vi "TL_stop_scan.vi"(5 "queue DAQ":refnum<queue>, 7 "queue sCMOS":refnum<queue>, 8 "error in":errorcluster, 9 "BF?":bool, 10 "queue piezo":refnum<queue>, 11 "queue ASI stage":refnum<queue>) -> (0 "error out":errorcluster)   [LabVIEW 2015]
uses:
  CONTROLS/Q_ASI_stage_element.ctl
  CONTROLS/Q_DAQ_element.ctl
  CONTROLS/Q_MCL_piezo_element.ctl
  CONTROLS/Q_camera_element.ctl
  GLOBAL/Global_DAQ.vi
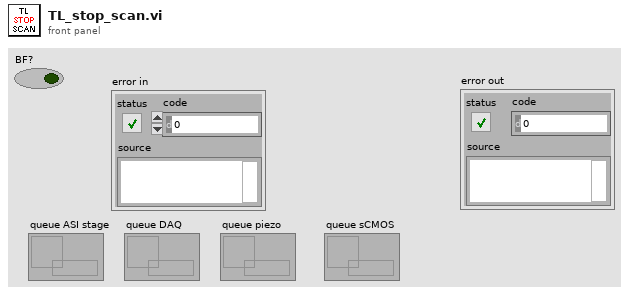
[diagram p1: front panel]
types:
  T1 = typedef "Q_camera_element.ctl" = cluster{"variant":variant, "Instruction":enum16{"CAMERA_idle", "CAMERA_initialize", "CAMERA_error", "CAMERA_security_stop", "CAMERA_not_acquiring", "CAMERA_acquiring", "CAMERA_start_acquiring", "CAMERA_stop_acquiring", "CAMERA_change_exposure", "CAMERA_define_ROI", "CAMERA_cooler", "CAMERA_acquire_movie", "CAMERA_init_scan", "CAMERA_check_new_scan_image", "CAMERA_close_scan", "CAMERA_init_merFISH", "CAMERA_start_acquiring_merFISH", "CAMERA_close_scan_merFISH", "CAMERA_close_merFISH", "CAMERA_init_TL", "CAMERA_start_acquiring_TL", "CAMERA_stop_acquiring_TL", "CAMERA_close_TL", "CAMERA_STOP"}}
  T2 = typedef "Q_MCL_piezo_element.ctl" = cluster{"variant":variant, "Instruction":enum16{"Piezo_idle", "Piezo_initialize", "Piezo_error", "Piezo_security_stop", "Piezo_read_z", "Piezo_move_z", "Piezo_keyboard_move", "Piezo_close_autofocus_calibration_ramp", "Piezo_change_init_state", "Piezo_init_autofocus", "Piezo_init_autofocus_merFISH_TL", "Piezo_autofocus", "Piezo_autofocus_merFISH_TL", "Piezo_stop_autofocus", "Piezo_stop_autofocus_merFISH_TL", "Piezo_autofocus_lost", "Piezo_resume_autofocus_merFISH_TL", "Piezo_check_z_position_merFISH_TL", "Piezo_init_ramp", "Piezo_move_z_ramp", "Piezo_close_ramp", "Piezo_close_merFISH", "Piezo_init_TL", "Piezo_close_ramp_TL", "Piezo_close_TL", "Piezo_stop"}}
  T3 = typedef "Q_ASI_stage_element.ctl" = cluster{"variant":variant, "Instruction":enum16{"ASI_idle", "ASI_initialize", "ASI_error", "ASI_security_stop", "ASI_read_XYZ", "ASI_up", "ASI_down", "ASI_left", "ASI_right", "ASI_save_XY", "ASI_move_to_XY", "ASI_brightfield", "ASI_init_scan", "ASI_init_merFISH", "ASI_move_to_XY_merFISH", "ASI_move_to_Z_merFISH", "ASI_init_autofocus_search_merFISH", "ASI_close_autofocus_search_merFISH", "ASI_adjust_piezo_autofocus_merFISH", "ASI_set_piezo_autofocus_to_reference_position_merFISH_TL", "ASI_close_merFISH", "ASI_init_TL", "ASI_move_mosaic_TL", "ASI_brightfield_TL", "ASI_close_TL", "ASI_stop"}}
  T4 = typedef "Q_DAQ_element.ctl" = cluster{"variant":variant, "Instruction":enum16{"DAQ_idle", "DAQ_initialize", "DAQ_error", "DAQ_security_stop", "DAQ_start_QPD", "DAQ_change_QPD_display", "DAQ_read_display_QPD_signal", "DAQ_QPD_init_autofocus", "DAQ_read_display_send_QPD_signal", "DAQ_close_autofocus_calibration_ramp", "DAQ_close_autofocus", "DAQ_405", "DAQ_488", "DAQ_561", "DAQ_641", "DAQ_zero_all", "DAQ_init_single_scan", "DAQ_single_scan", "DAQ_two_way_valve", "DAQ_init_merFISH", "DAQ_scan_merFISH", "DAQ_photobleaching_merFISH", "DAQ_close_merFISH", "DAQ_init_TL", "DAQ_synchro_TL", "DAQ_close_task_TL", "DAQ_close_TL", "DAQ_stop"}}
  T5 = enum16{"DAQ_idle", "DAQ_initialize", "DAQ_error", "DAQ_security_stop", "DAQ_start_QPD", "DAQ_change_QPD_display", "DAQ_read_display_QPD_signal", "DAQ_QPD_init_autofocus", "DAQ_read_display_send_QPD_signal", "DAQ_close_autofocus_calibration_ramp", "DAQ_close_autofocus", "DAQ_405", "DAQ_488", "DAQ_561", "DAQ_641", "DAQ_zero_all", "DAQ_init_single_scan", "DAQ_single_scan", "DAQ_two_way_valve", "DAQ_init_merFISH", "DAQ_scan_merFISH", "DAQ_photobleaching_merFISH", "DAQ_close_merFISH", "DAQ_init_TL", "DAQ_synchro_TL", "DAQ_close_task_TL", "DAQ_close_TL", "DAQ_stop"}
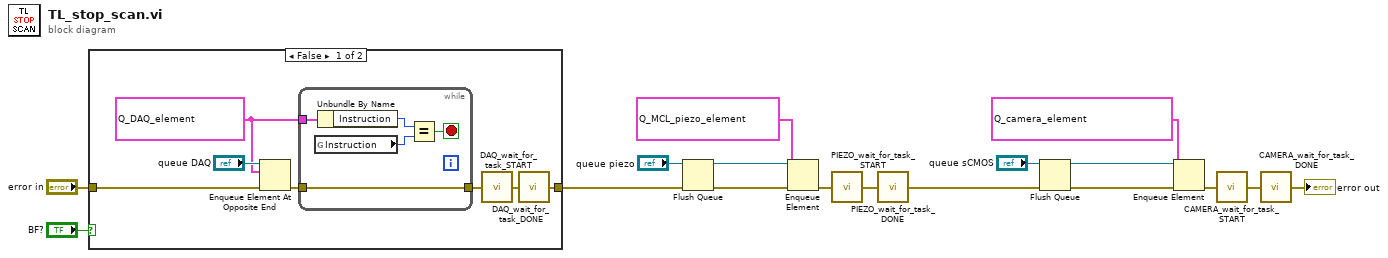
[diagram p0: block diagram]
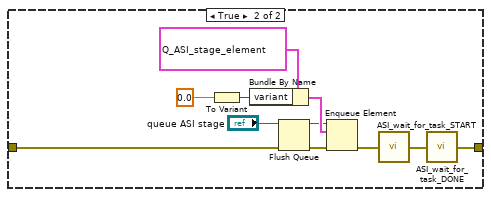
[diagram p2: hidden frame]
diagram:
  n1 = case shown="False" "BF?" {
    tunnel: "error in" -> [w24 w33]
    tunnel: [w22 w37] -> w14
    frame False {
      w18 = T4 {"variant"=variant, "Instruction"=enum."DAQ_close_task_TL"} ("Q_DAQ")
      n2 = Enqueue Element At Opposite End(queue="queue DAQ", element=w18, error in (no error)=w24) -> (error out=w20:errorcluster)  [unwired: 1 in, 2 out]
      n3 = while {
        tunnel: w20 -> [w26]
        tunnel: [w26] -> w19
        tunnel: w18 -> [w25]
        stop <- w28 stop-if-true
        n4 = global read "Global_DAQ.vi" "Instruction"() -> (w29:T5)
        n5 = Unbundle By Name(w25) -> ("Instruction"=w27:T5)
        n6 = Equal?(x=w27, y=w29) -> (x = y?=w28:bool)
      }
      n7 = call "DAQ_wait_for_task_START.vi"("error in"=w19) -> ("error out"=w23:errorcluster)
      n8 = call "DAQ_wait_for_task_DONE.vi"("error in"=w23) -> ("error out"=w22:errorcluster)
    }
    frame True {
      n9 = To Variant(anything=0.0) -> (Variant=w38:variant)
      n10 = Bundle By Name(cluster=T3 {"variant"=variant, "Instruction"=enum."ASI_brightfield_TL"} ("element"), "variant"=w38) -> (w34:T3)
      n11 = Flush Queue(queue="queue ASI stage", error in (no error)=w33) -> (queue out=w30:refnum<queue>, error out=w32:errorcluster)  [unwired: 1 out]
      n12 = Enqueue Element(queue=w30, element=w34, error in (no error)=w32) -> (error out=w39:errorcluster)  [unwired: 1 in, 2 out]
      n13 = call "ASI_wait_for_task_START.vi"("error in"=w39) -> ("error out"=w40:errorcluster)
      n14 = call "ASI_wait_for_task_DONE.vi"("error in"=w40) -> ("error out"=w37:errorcluster)
    }
  }
  n15 = Flush Queue(queue="queue piezo", error in (no error)=w14) -> (queue out=w12:refnum<queue>, error out=w15:errorcluster)  [unwired: 1 out]
  n16 = Enqueue Element(queue=w12, element=T2 {"variant"=variant, "Instruction"=enum."Piezo_close_ramp_TL"}, error in (no error)=w15) -> (error out=w10:errorcluster)  [unwired: 1 in, 2 out]
  n17 = call "PIEZO_wait_for_task_START.vi"("error in"=w10) -> ("error out"=w9:errorcluster)
  n18 = call "PIEZO_wait_for_task_DONE.vi"("error in"=w9) -> ("error out"=w7:errorcluster)
  n19 = Flush Queue(queue="queue sCMOS", error in (no error)=w7) -> (queue out=w5:refnum<queue>, error out=w8:errorcluster)  [unwired: 1 out]
  n20 = Enqueue Element(queue=w5, element=T1 {"variant"=variant, "Instruction"=enum."CAMERA_stop_acquiring_TL"}, error in (no error)=w8) -> (error out=w3:errorcluster)  [unwired: 1 in, 2 out]
  n21 = call "CAMERA_wait_for_task_START.vi"("error in"=w3) -> ("error out"=w2:errorcluster)
  n22 = call "CAMERA_wait_for_task_DONE.vi"("error in"=w2) -> ("error out"=→"error out":errorcluster)
